vi "SuperAuton-NoPullOff.vi"(8 "error in (no error)":errorcluster, 9 "TimeToPull":dbl, 11 "Auton Event Queue Data":refnum<queue>) -> (0 "error out":errorcluster, 2 "Success?":bool, 3 "Auton Event Queue Data 2":refnum<queue>)   [LabVIEW 2014]
uses:
  Robot Global Data.vi
  <vilib>/Rock Robotics/WPI/RobotDrive/WPI_RobotDriveGetSetRefNum.vi
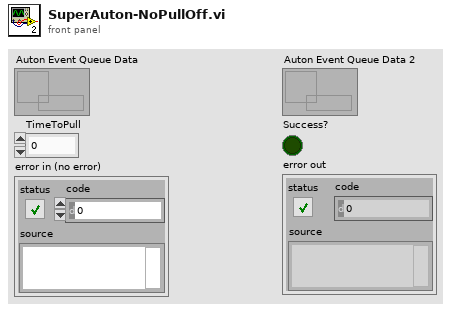
[diagram p1: front panel]
types:
  T1 = typedef "WPI_RobotDriveDevRef.ctl" = cluster{"DevStatus":errorcluster, "Motors[]":T2[], "Square Inputs":bool, "Max Output":dbl}
  T2 = typedef "WPI_MotorControlDeviceRef.ctl" = cluster{"DeviceStatus":errorcluster, "Type":T3, "PWM":cluster{"Controller":T4, "PWM Channel":T5, "DeadBand":T6}, "CAN":cluster{"Device Number":u8, "Control Mode":T7, "Semaphore":T8, "Max Vout":dbl, "TalonSRX Control Mode":T9}, "Invert":bool, "TransformRef":T10, "InvTransformRef":T10}
  T3 = typedef "WPI_MotorControlType.ctl" = enum16{"PWM", "CAN", "CANTalonSRX"}
  T4 = typedef "FPGA_TypedefDigitalModule.ctl" = enum16{"Controller 1"}
  T5 = typedef "FPGA_DIOPWMChannel.ctl" = enum8{"PWM 0", "PWM 1", "PWM 2", "PWM 3", "PWM 4", "PWM 5", "PWM 6", "PWM 7", "PWM 8", "PWM 9", "PWM MXP 0", "PWM MXP 1", "PWM MXP 2", "PWM MXP 3", "PWM MXP 4", "PWM MXP 5", "PWM MXP 6", "PWM MXP 7", "PWM MXP 8", "PWM MXP 9", "Invalid"}
  T6 = typedef "WPI_PWMDeadband.ctl" = cluster{"Name":string, "maxPositivePwm":i32, "minPositivePwm":i32, "centerPwm":i32, "maxNegativePwm":i32, "minNegativePwm":i32, "angularRange":u16}
  T7 = typedef "WPI_CANJaguar_ControlMode.ctl" = enum8{"Percent VBus", "Current", "Speed", "Position", "Voltage"}
  T8 = typedef "Semaphore RefNum" = refnum<k1>
  T9 = typedef "WPI_CANTalonSRX_APIControlMode.ctl" = enum8{"Percent VBus", "Speed", "Position", "Slave", "Unchanged / Invalid"}
  T10 = typedef "WPI_PWMTransform_ConPane.ctl" = refnum<vi>
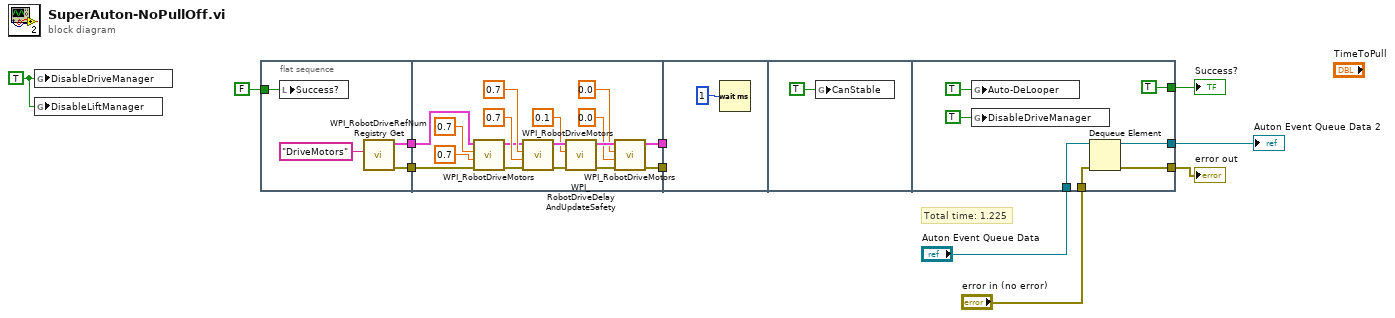
[diagram p0: block diagram]
diagram:
  w7 = TRUE ("Success?")
  # "Total time: 1.225"
  n1 = global write "Robot Global Data.vi" "DisableDriveManager"(w7) -> ()
  n2 = global write "Robot Global Data.vi" "DisableLiftManager"(w7) -> ()
  n3 = flat-sequence {
    tunnel: FALSE ("Success?") -> [w15]
    tunnel: [w13] -> w5
    tunnel: [w12] -> w6
    tunnel: w6 -> [w18]
    tunnel: w5 -> [w19]
    tunnel: [w32] -> w4
    tunnel: [w31] -> w3
    tunnel: w4 -> [_]
    tunnel: w3 -> [_]
    tunnel: [TRUE ("Success?")] -> w2
    tunnel: "Auton Event Queue Data" -> [w38]
    tunnel: "error in (no error)" -> [w37]
    tunnel: [w36] -> w9
    tunnel: [w35] -> w8
    frame #0 {
      n4 = local write "Success?"(w15) -> ()
      n5 = call <vilib>:"WPI_RobotDriveRefNum Registry Get.vi"("refnum name"="DriveMotors") -> ("error out"=w12:errorcluster, "RobotDriveDevRef"=w13:T1)  [unwired: 9 in]
    }
    frame #1 {
      n6 = call <vilib>:"WPI_RobotDriveMotors.vi"("error in (no error)"=w18, "RightSpeed"=0.7 ("Y axis value"), "LeftSpeed"=0.7 ("X axis value"), "RobotDriveDevRef"=w19) -> ("error out"=w16:errorcluster, "RobotDriveDevRef"=w17:T1)  [unwired: 5 in, 1 out]
      n7 = call <vilib>:"WPI_RobotDriveMotors.vi"("error in (no error)"=w16, "RightSpeed"=0.7 ("Y axis value"), "LeftSpeed"=0.7 ("X axis value"), "RobotDriveDevRef"=w17) -> ("error out"=w27:errorcluster, "RobotDriveDevRef"=w28:T1)  [unwired: 5 in, 1 out]
      n8 = call <vilib>:"WPI_RobotDriveDelayAndUpdateSafety.vi"("error in (no error)"=w27, "Delay (s)"=0.1, "RobotDriveDevRef"=w28) -> ("error out"=w24:errorcluster, "RobotDriveDevRef 2"=w25:T1)  [unwired: 7 in]
      n9 = call <vilib>:"WPI_RobotDriveMotors.vi"("error in (no error)"=w24, "RightSpeed"=0.0 ("Y axis value"), "LeftSpeed"=0.0 ("X axis value"), "RobotDriveDevRef"=w25) -> ("error out"=w31:errorcluster, "RobotDriveDevRef"=w32:T1)  [unwired: 5 in, 1 out]
    }
    frame #2 {
      n10 = Wait (ms)(milliseconds to wait=u32 1) -> ()  [unwired: 1 out]
    }
    frame #3 {
      n11 = global write "Robot Global Data.vi" "CanStable"(TRUE) -> ()
    }
    frame #4 {
      n12 = global write "Robot Global Data.vi" "Auto-DeLooper"(TRUE ("DisableDriveManager")) -> ()
      n13 = global write "Robot Global Data.vi" "DisableDriveManager"(TRUE ("DisableDriveManager")) -> ()
      n14 = Dequeue Element(queue=w38, error in (no error)=w37) -> (queue out=w36:refnum<queue>, error out=w35:errorcluster)  [unwired: 1 in, 2 out]
    }
  }
  "error out" <- w8
  "Auton Event Queue Data 2" <- w9
  "Success?" <- w2
